vi "Flow Rate Calculator.vi"() -> ()   [LabVIEW 2015]
doc: "Example VI that demonstrates all library features."
uses:
  PL GCF Calculator.lvlib
panel:
  out "error":bool
  out "actual gas flow rate":dbl
  in  "actual gas/mixture":string(combo)="Ar"
  in  "calibration gas":string(combo)="N2"
  in  "GCF data source":u16(ring) items=["Bronkhorst", "Brooks", "MKS"]
  in  "measured gas flow rate":dbl
  # "Mixture string example:\n\"80% Ar + 20% O2\"."
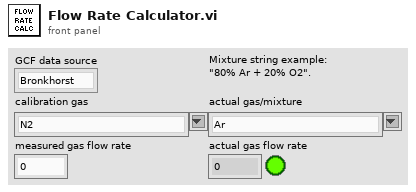
[diagram p1: front panel]
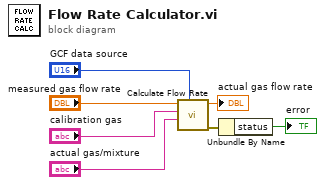
[diagram p0: block diagram]
diagram:
  n1 = call "Calculate Flow Rate.vi"("GCF data source (Bronkhorst)"="GCF data source", "actual gas/mixture"="actual gas/mixture", "calibration gas"="calibration gas", "measured gas flow rate"="measured gas flow rate") -> ("error out"=w2:errorcluster, "actual gas flow rate"=→"actual gas flow rate":dbl)  [unwired: 6 in]
  n2 = Unbundle By Name(w2) -> ("status"=→"error":bool)
